vi "ARC_Queue Create_Array.vi"(8 "error in (no error)":errorcluster caption="Error In (no error)", 10 "Max Queue Size(-1)":i32=-1, 11 "Queue Array":string[](array[string])) -> (0 "error out":errorcluster caption="Error Out", 2 "Creat New?":bool[](array[boolean]))   [LabVIEW 2016]
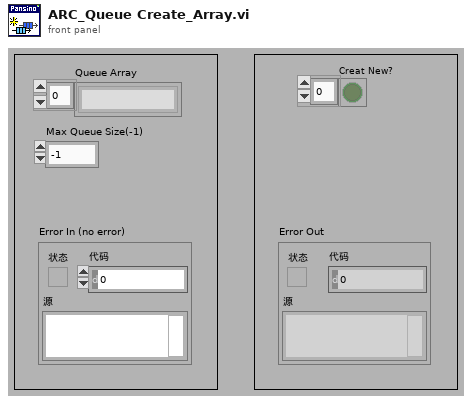
[diagram p1: front panel]
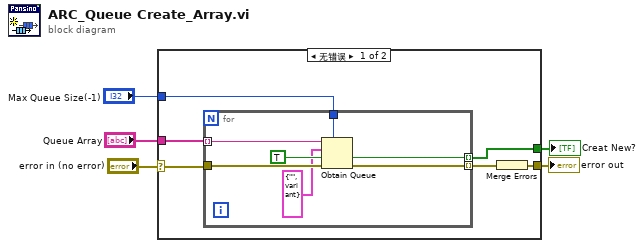
[diagram p0: block diagram]
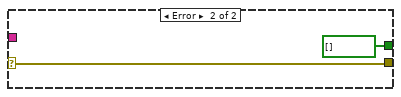
[diagram p2: hidden frame]
diagram:
  n1 = case shown="无错误" "error in (no error)" {
    selector: "error in (no error)" -> [w11 w20]
    tunnel: [w9 w20] -> w4
    tunnel: "Max Queue Size(-1)" -> [w8 _]
    tunnel: "Queue Array" -> [w7 _]
    tunnel: [w6 bool[] []] -> w1
    frame No Error {
      n2 = for {
        tunnel: w8 -> [w15]
        tunnel: w7 -> [w16] mode=indexing
        tunnel: [w14] -> w6 mode=indexing
        tunnel: w11 -> [w18]
        tunnel: [w17] -> w10 mode=indexing
        n3 = Obtain Queue(max queue size (-1, unlimited)=w15, name (unnamed)=w16, element data type=cluster{"Event":string, "Data":variant} {"Event"="", "Data"=variant} ("输出簇"), create if not found? (T)=TRUE ("如未找到是否创建？(T)"), error in (no error)=w18) -> (created new?=w14:bool, error out=w17:errorcluster)  [unwired: 1 out]
      }
      n4 = Merge Errors(w10) -> (w9:errorcluster)
    }
    frame Error {
    }
  }
  "error out" <- w4
  "Creat New?" <- w1
